vi "SimpleBallPlacementAllyRole.vi"(7 "first call":bool, 8 "error in (no error)":errorcluster, 9 "Tactic index in":i32, 10 "Game in":refnum<class "Game.lvclass">, 11 "SimpleBallPlacementAllyRole in":refnum<class "SimpleBallPlacementAllyRole.lvclass">) -> (0 "error out":errorcluster, 1 "tactic index":i32, 2 "Robot out":refnum<class "Robot.lvclass">, 3 "SimpleBallPlacementAllyRole out":refnum<class "SimpleBallPlacementAllyRole.lvclass">)   [LabVIEW 2020, in "SimpleBallPlacementAllyRole.lvclass"]
uses:
  SimpleBallPlacementAllyRole.lvclass
  C:/RoboIME/SSL_AI/Role_class/Role.lvclass
  Game_class/Game.lvclass
  Robot_class/Robot.lvclass
  Role_class/Role.lvclass/Role.ctl
  SimpleBallPlacementAllyRole.lvclass/SimpleBallPlacementAllyRole.ctl
  Tacticbook_class/Tacticbook.lvclass/Tacticbook.ctl
  GoToBallPlacementAllyTactic_class/GoToBallPlacementAllyTactic.lvclass/GoToBallPlacementAllyTactic.ctl
  PlaceBallTactic_class/PlaceBallTactic.lvclass/PlaceBallTactic.ctl
  Tacticbook_class/Read GoToBallPlacementAllyTactic.vi
  GoToBallPlacementAllyTactic_class/Read States.vi
  Tacticbook_class/Write GoToBallPlacementAllyTactic.vi
  Tacticbook_class/Read PlaceBallTactic.vi
  PlaceBallTactic_class/Read States.vi
  Tacticbook_class/Write PlaceBallTactic.vi
  Role_class/Read Tacticbook.vi
  Read number_of_tactics.vi
  Role_class/Write Tacticbook.vi
  Role_class/Write tactic_index.vi
  Role_class/Read RobotRef.vi
  Tacticbook_class/Tacticbook.lvclass
  GoToBallPlacementAllyTactic_class/GoToBallPlacementAllyTactic.lvclass
  PlaceBallTactic_class/PlaceBallTactic.lvclass
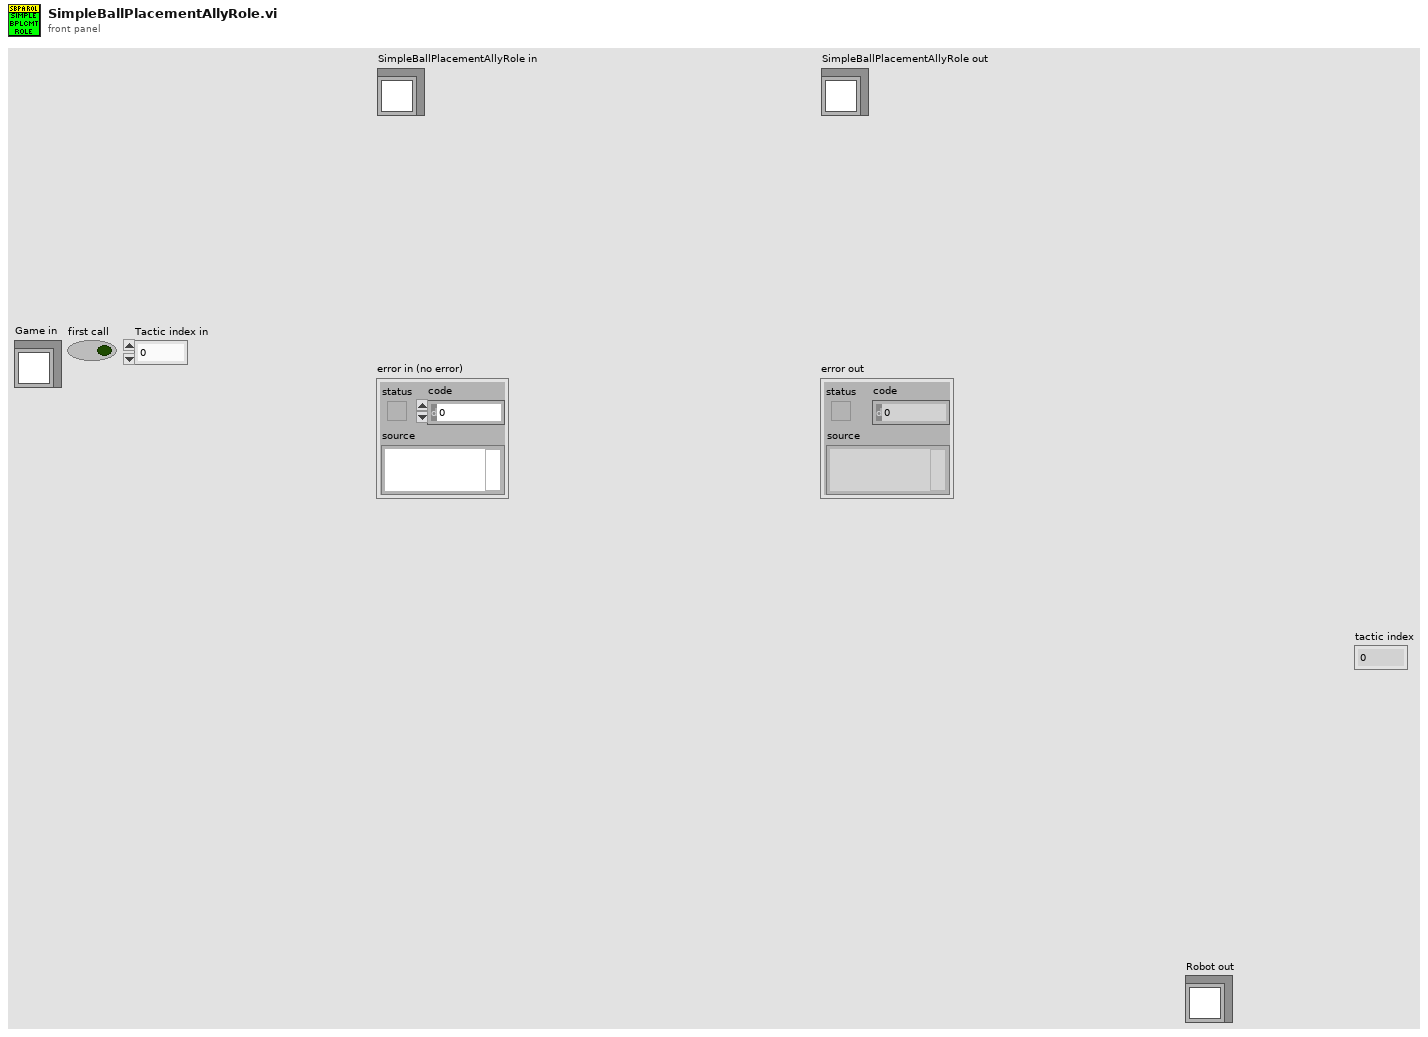
[diagram p1: front panel]
types:
  T1 = typedef "StatesGoToBallPlacementAllyTactic.ctl" = enum16{"GoToNearBall", "GoToBall", "PrepareToPositionBall", "Exit"}
  T2 = typedef "StatesPlaceBallTactic.ctl" = enum16{"GoToGetBall", "PlaceBall", "Exit"}
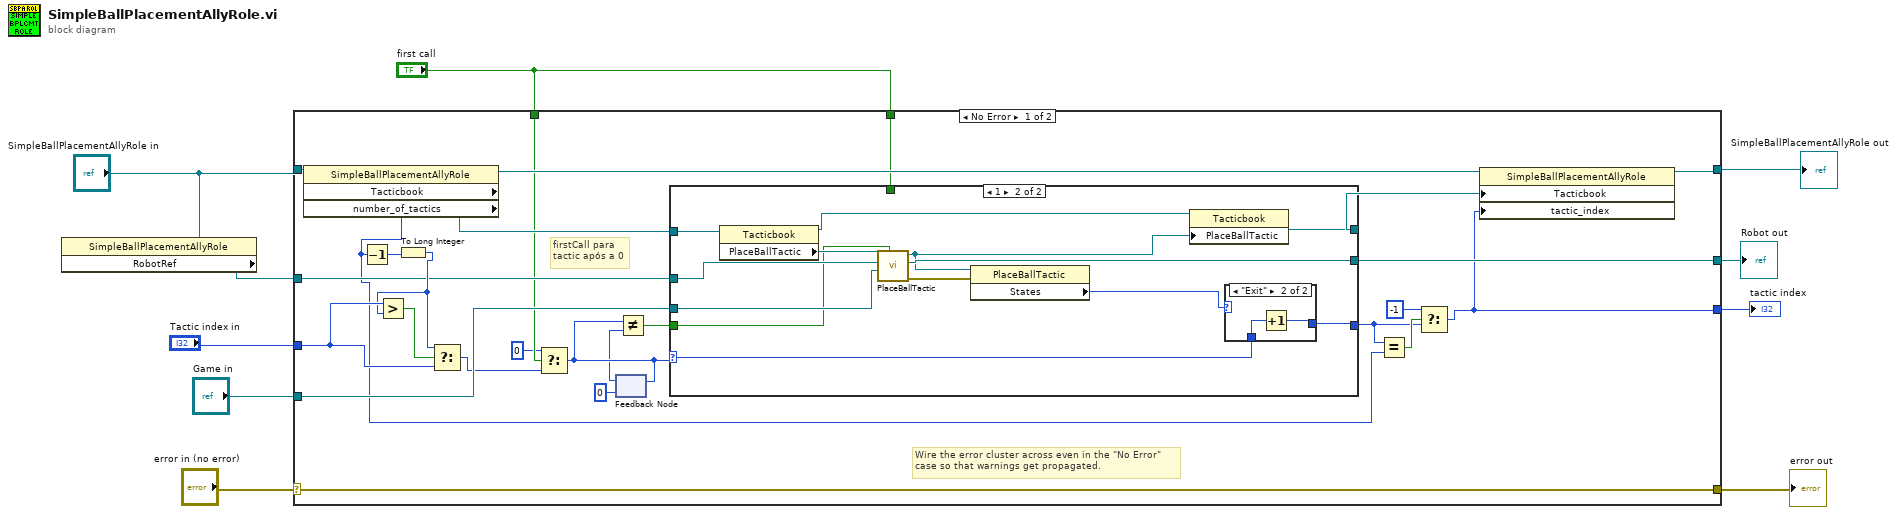
[diagram p0: block diagram]
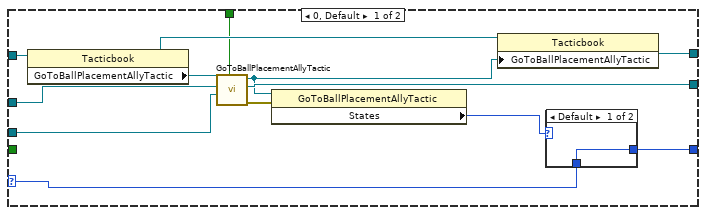
[diagram p2: hidden frame]
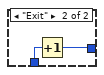
[diagram p3: hidden frame]
diagram:
  n1 = property class="SimpleBallPlacementAllyRole"(reference="SimpleBallPlacementAllyRole in") -> ("RobotRef"=w9:refnum<class "Robot.lvclass">)  [unwired: 1 in, 2 out]
  n2 = case shown="No Error" "error in (no error)" {
    selector: "error in (no error)" -> [w36 w71]
    tunnel: [w36 w71] -> w5
    tunnel: [w34 w70] -> w2
    tunnel: "SimpleBallPlacementAllyRole in" -> [w35 w70]
    tunnel: w9 -> [w24 w69]
    tunnel: [w23 w69] -> w7
    tunnel: "Game in" -> [w30 _]
    tunnel: [w13 _] -> w6
    tunnel: "Tactic index in" -> [w28 _]
    tunnel: "first call" -> [w27 _]
    tunnel: "first call" -> [w22 _]
    frame No Error {
      # "firstCall para\ntactic após a 0"
      # "Wire the error cluster across even in the \"No Error\"\ncase so that warnings get propagated."
      n3 = property class="SimpleBallPlacementAllyRole"(reference=w35) -> (reference out=w33:refnum<class "SimpleBallPlacementAllyRole.lvclass">, "Tacticbook"=w32:refnum<class "Tacticbook.lvclass">, "number_of_tactics"=w11:u32)  [unwired: 1 in, 1 out]
      n4 = Decrement(x=w11) -> (x-1=w26:u32)
      n5 = To Long Integer(number=w26) -> (32bit integer=w25:i32)
      n6 = Greater?(x=w28, y=w25) -> (0:w29:bool)
      n7 = Select(t=w25, s=w29, f=w28) -> (s? t:f=w21:i32)
      n8 = Select(t=0, s=w22, f=w21) -> (s? t:f=w19:i32)
      n9 = feedback-in #1(w19) -> ()
      n10 = feedback #1(0 ("Tactic index in")) -> (w18:i32)
      n11 = Not Equal?(x=w19, y=w18) -> (x != y?=w16:bool)
      n12 = case shown="1" w19 {
        selector: w19 -> [w38 w54]
        tunnel: [w46 w55] -> w14
        tunnel: w32 -> [w49 w65]
        tunnel: w24 -> [w42 w60]
        tunnel: [w47 w63] -> w31
        tunnel: w30 -> [w41 w59]
        tunnel: w27 -> [w44 _]
        tunnel: [w40 w58] -> w23
        tunnel: w16 -> [_ w56]
        frame 0, Default {
          n13 = property class="Tacticbook"(reference=w49) -> (reference out=w48:refnum<class "Tacticbook.lvclass">, "GoToBallPlacementAllyTactic"=w43:refnum<class "GoToBallPlacementAllyTactic.lvclass">)  [unwired: 1 in, 1 out]
          n14 = call "GoToBallPlacementAllyTactic.vi"("firstCall"=w44, "Game in"=w41, "Robot"=w42, "GoToBallPlacementAllyTactic in"=w43) -> ("error out"=w45:errorcluster, "Robot out"=w40:refnum<class "Robot.lvclass">, "GoToBallPlacementAllyTactic out"=w39:refnum<class "GoToBallPlacementAllyTactic.lvclass">)  [unwired: 5 in]
          n15 = property class="GoToBallPlacementAllyTactic"(reference=w39, error in=w45) -> ("States"=w37:T1)  [unwired: 2 out]
          n16 = property class="Tacticbook"(reference=w48, "GoToBallPlacementAllyTactic"=w39) -> (reference out=w47:refnum<class "Tacticbook.lvclass">)  [unwired: 1 in, 1 out]
          n17 = case shown="Default" w37 {
            tunnel: [w50 w52] -> w46
            tunnel: w38 -> [w50 w51]
            frame Default {
            }
            frame "Exit" {
              n18 = Increment(x=w51) -> (x+1=w52:i32)
            }
          }
        }
        frame 1 {
          n19 = property class="Tacticbook"(reference=w65) -> (reference out=w64:refnum<class "Tacticbook.lvclass">, "PlaceBallTactic"=w61:refnum<class "PlaceBallTactic.lvclass">)  [unwired: 1 in, 1 out]
          n20 = call "PlaceBallTactic.vi"("firstCall"=w56, "Game in"=w59, "Robot"=w60, "PlaceBallTactic in"=w61) -> ("error out"=w62:errorcluster, "Robot out"=w58:refnum<class "Robot.lvclass">, "PlaceBallTactic out"=w57:refnum<class "PlaceBallTactic.lvclass">)  [unwired: 5 in]
          n21 = property class="PlaceBallTactic"(reference=w57, error in=w62) -> ("States"=w53:T2)  [unwired: 2 out]
          n22 = property class="Tacticbook"(reference=w64, "PlaceBallTactic"=w57) -> (reference out=w63:refnum<class "Tacticbook.lvclass">)  [unwired: 1 in, 1 out]
          n23 = case shown="\"Exit\"" w53 {
            tunnel: [w66 w68] -> w55
            tunnel: w54 -> [w66 w67]
            frame Default {
            }
            frame "Exit" {
              n24 = Increment(x=w67) -> (x+1=w68:i32)
            }
          }
        }
      }
      n25 = Equal?(x=w14, y=w11) -> (x = y?=w15:bool)
      n26 = Select(t=-1, s=w15, f=w14) -> (s? t:f=w13:i32)
      n27 = property class="SimpleBallPlacementAllyRole"(reference=w33, "Tacticbook"=w31, "tactic_index"=w13) -> (reference out=w34:refnum<class "SimpleBallPlacementAllyRole.lvclass">)  [unwired: 1 in, 1 out]
    }
    frame Error {
    }
  }
  "error out" <- w5
  "SimpleBallPlacementAllyRole out" <- w2
  "Robot out" <- w7
  "tactic index" <- w6
